vi "Get AnotherChild.vi"(8 "error in (no error)":errorcluster caption="错误输入（无错误）", 10 "ChildNode*":refnum<data-value>, 11 "PanelLinkNode 输入":refnum<class "PanelLinkNode.lvclass"> caption="DNL_LabVIEW Object in") -> (0 "error out":errorcluster caption="错误输出", 2 "AnotherChildNode*":refnum<data-value>, 3 "PanelLinkNode 输出":refnum<class "PanelLinkNode.lvclass"> caption="DNL_LabVIEW Object out")   [LabVIEW 2016, in "PanelLinkNode.lvclass"]
uses:
  PanelLinkNode.lvclass
  PanelObject/PanelObject.lvclass
  PanelLinkNode.lvclass/PanelLinkNode.ctl
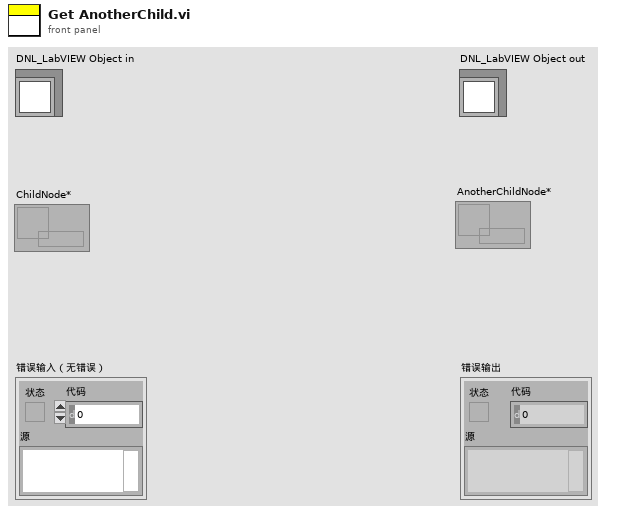
[diagram p1: front panel]
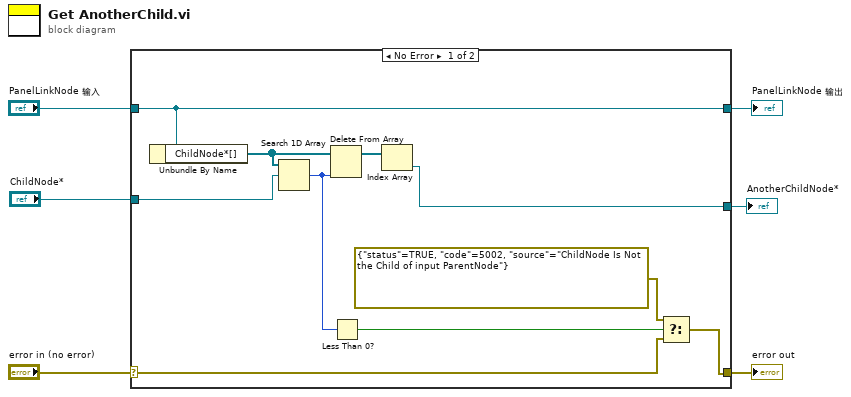
[diagram p0: block diagram]
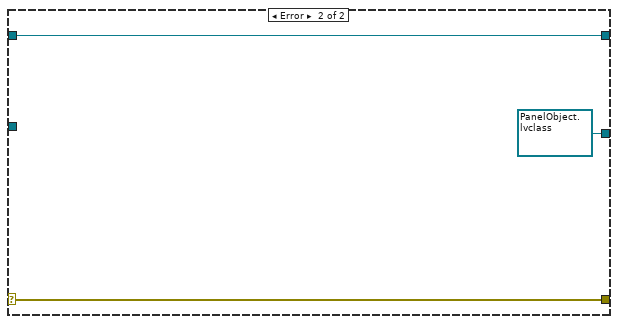
[diagram p2: hidden frame]
diagram:
  n1 = case shown="No Error" "error in (no error)" {
    selector: "error in (no error)" -> [w8 w19]
    tunnel: [w7 w19] -> w5
    tunnel: [w15 w18] -> w3
    tunnel: "PanelLinkNode 输入" -> [w15 w18]
    tunnel: "ChildNode*" -> [w13 _]
    tunnel: [w12 refnum<data-value> refnum ("ChildNode*")] -> w1
    frame No Error {
      n2 = Unbundle By Name(w15) -> ("ChildNode*[]"=w14:refnum<data-value>[])
      n3 = Search 1D Array(1D array=w14, element=w13) -> (index of element=w11:i32)  [unwired: 1 in]
      n4 = Delete From Array(array=w14, index=w11) -> (array with subset deleted=w16:refnum<data-value>[])  [unwired: 1 in, 1 out]
      n5 = Less Than 0?(x=w11) -> (x < 0?=w9:bool)
      n6 = Index Array(array=w16) -> (element=w12:refnum<data-value>)  [unwired: 1 in]
      n7 = Select(t=errorcluster {"status"=TRUE, "code"=5002, "source"="ChildNode Is Not the Child of input ParentNode"} ("错误常量"), s=w9, f=w8) -> (s? t:f=w7:errorcluster)
    }
    frame Error {
    }
  }
  "error out" <- w5
  "PanelLinkNode 输出" <- w3
  "AnotherChildNode*" <- w1
